vi "main_120MHz.vi"() -> ()   [LabVIEW 2010]
uses:
  <vilib>/Platform/TimedLoop/XDataNode/XDataNode.xnode
  <vilib>/Platform/TimedLoop/XDataNode/nitl_modes.ctl
  <vilib>/Platform/TimedLoop/XDataNode/XDNodeRunTimeDep.lvlib
  <vilib>/Platform/TimedLoop/XDataNode/wakeup.ctl
  <vilib>/Platform/TimedLoop/XDataNode/timing_clust.ctl
  <vilib>/eio/EIONode/EIONode.xnode
  common_typedefs/channels_cluster.ctl
  common_typedefs/gate_parameters_cluster.ctl
panel:
  in  "clamp first pixel?":bool
  in  "gate 3":T1
  in  "gate 2":T1
  in  "gate 1":T1
  out "integrated pixel values":T2
  out "data read":T2
  in  "channel offsets":T2
  out "clock 3 state":bool
  out "clock 2 state":bool
  out "clock 1 state":bool
  in  "stop acquisition at FIFO overflow?":bool=TRUE
  in  "wait for trigger?":bool
  in  "stop":bool
  in  "acquire":bool
  out "acquiring?":bool
  out "FIFO overflow":bool
  out "current pixel no.":i64
  in  "number of pixels":i64=-1
  in  "maximum bit depth":i8
  in  "iterations per pixel":u32
  in  "enable ADC clock?":bool=TRUE
  in  "ADC clock phase":u8
  in  "converter box version":i16=1 min=1 max=2
  # "Outputs / displays"
  # "Integration parameters"
  # "Clock parameters"
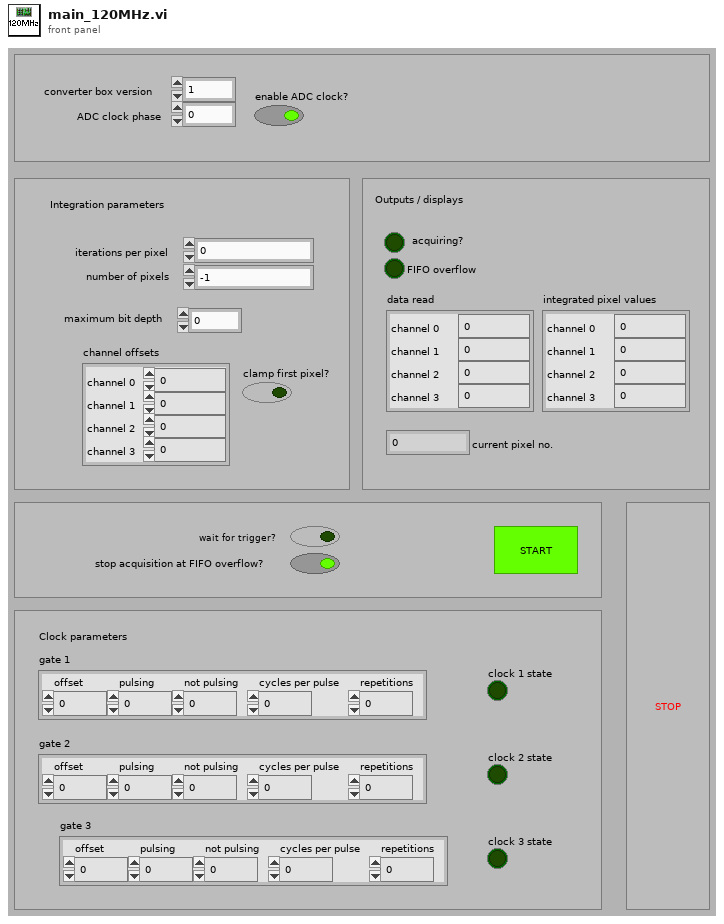
[diagram p1: front panel]
types:
  T1 = typedef "gate_parameters_cluster.ctl" = cluster{"offset":i64, "pulsing":i64, "not pulsing":i64, "cycles per pulse":i64, "repetitions":i64}
  T2 = typedef "channels_cluster.ctl" = cluster{"channel 0":u32, "channel 1":u32, "channel 2":u32, "channel 3":u32}
  T3 = typedef "XDNodeRunTimeDep.lvlib/timing_clust.ctl" = cluster{"Expected End [f-1]":u64, "Actual End [f-1]":u64, "Finished Late? [f-1]":bool, "Expected End [i-1]":u64, "Actual End [i-1]":u64, "Finished Late? [i-1]":bool, "Expected Start [i]":u64, "Actual Start [i]":u64, "Expected Start [f]":u64, "Actual Start [f]":u64, "Source Name":string, "Structure Name":string, "Period":i64, "Deadline":i64, "Offset":i64, "Start":i64, "Priority":i32, "Timeout":i32, "Mode":T4, "Wakeup Reason":T5, "Error":errorcluster, "Source Type":string, "Secondary Source Type":string, "Global End Time":u64, "Global Start Time":u64, "Frame Duration":u64, "Iteration Duration":u64, "Assigned CPU":i32, "I/O Scan Engine Mode":u32}
  T4 = typedef "XDNodeRunTimeDep.lvlib/nitl_modes.ctl" = enum32{"No Change", "Process missed periods, maintain original phase", "Discard missed periods, maintain original phase", "Process missed periods, ignore original phase", "Discard missed periods, ignore original phase"}
  T5 = typedef "XDNodeRunTimeDep.lvlib/wakeup.ctl" = enum32{"Normal", "Aborted", "Asynchronous wakeup", "Timing source error", "Timed loop error", "Timeout"}
  T6 = typedef "gate_counters_cluster.ctl" = cluster{"phase iteration counter":i64, "phase repetition counter":i64, "pulse iteration counter":i64, "phase state":bool}
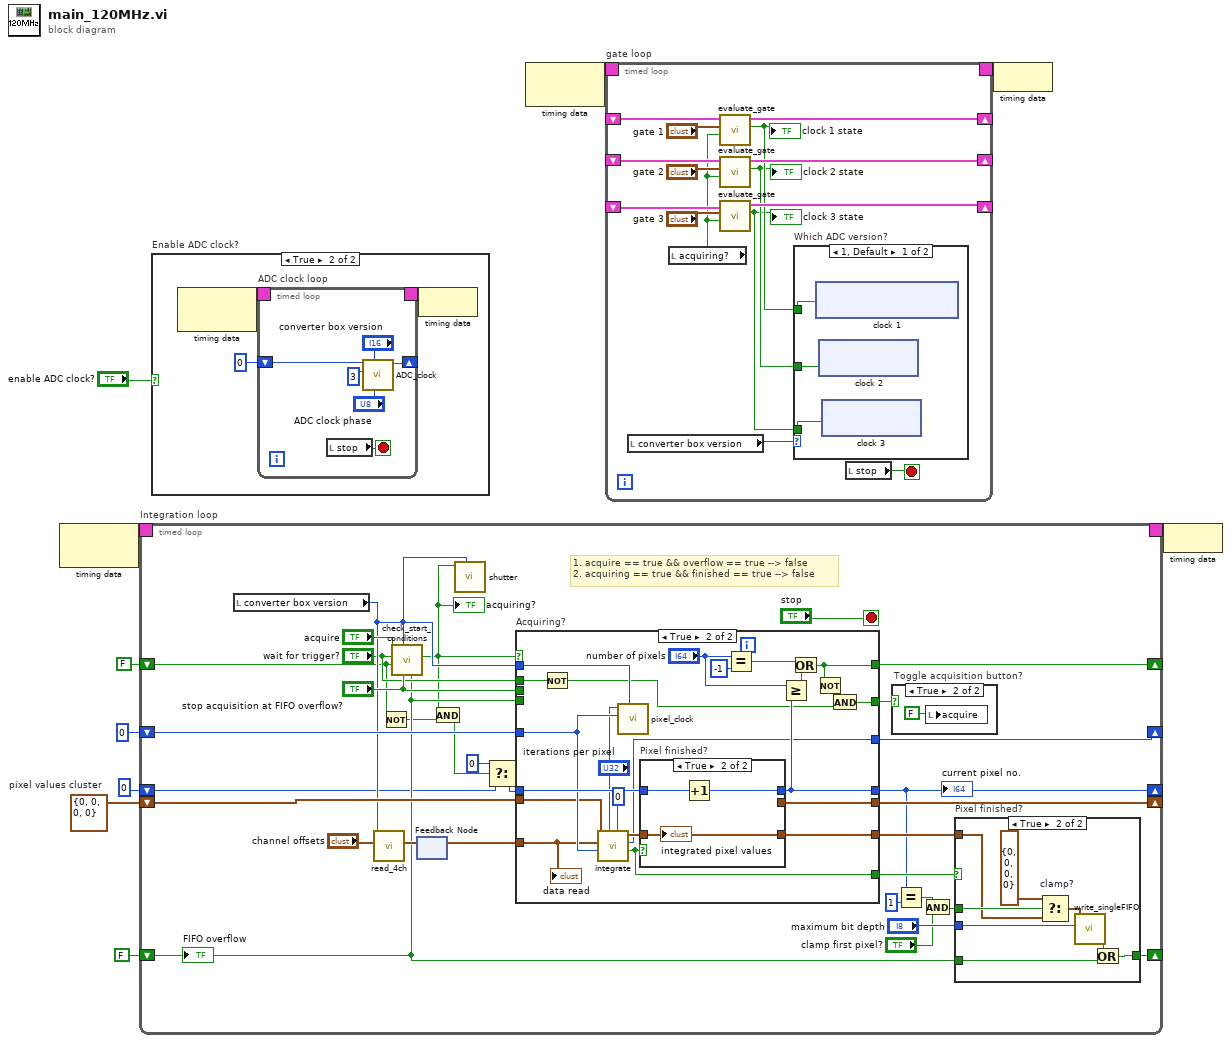
[diagram p0: block diagram]
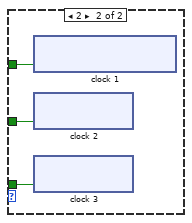
[diagram p2: hidden frame]
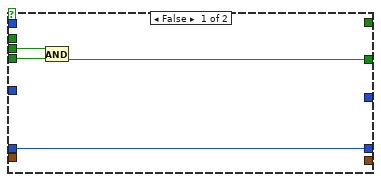
[diagram p5: hidden frame]
diagram:
  w4 = T2 {"channel 0"=0, "channel 1"=0, "channel 2"=0, "channel 3"=0}  # pixel values cluster
  n1 = node-c288() -> (w9:T3)  [unwired: 1 in]
  n2 = timed-loop "Integration loop" {
    timing: w9 -> [_]
    timing-out: [_] -> w8
    shift-right: [w18] -> _
    shift-left: i64 0 -> [w16]
    shift-right: [w36] -> _
    shift-left: u32 0 ("iteration counter out") -> [w38]
    shift-right: [w37] -> _
    shift-left: w4 -> [w39]
    shift-right: [w27] -> _
    shift-left: FALSE -> [w26]
    shift-right: [w31] -> _
    shift-left: FALSE -> [w12]
    stop <- "stop" stop-if-true
    # "1. acquire == true && overflow == true --> false\n2. acquiring == true && finished == true --> false"
    n3 = local read "converter box version"() -> (w30:i16)
    n4 = call "read_4ch.vi"("channel offsets"="channel offsets", "converter box version"=w30) -> ("read output"=w34:T2)  [unwired: 9 in]
    n5 = Not(x=w12) -> (.not. x?=w13:bool)
    n6 = call "check_start_conditions.vi"("FIFO overflow?"=w26, "stop at FIFO overflow?"="stop acquisition at FIFO overflow?", "converter box version"=w30, "already acquiring?"=w12, "in triggered mode?"="wait for trigger?", "acquire"="acquire") -> ("acquire?"=w11:bool)  [unwired: 5 in]
    "acquiring?" <- w11
    n7 = feedback-in #1(w34) -> ()
    n8 = feedback #1() -> (w33:T2)  [unwired: 1 in]
    n9 = And(x=w11, y=w13) -> (x .and. y?=w14:bool)
    n10 = call "shutter.vi"("converter box version"=w30, "open?"=w11) -> ()  [unwired: 10 in]
    n11 = Select(t=i64 0, s=w14, f=w16) -> (s? t:f=w15:i64)
    n12 = case "Acquiring?" shown="True" w11 {
      tunnel: w30 -> [_ w77]
      tunnel: [_ w63] -> w25
      tunnel: [_ w69] -> w36
      tunnel: [w52 w73] -> w18
      tunnel: w39 -> [_ w66]
      tunnel: w15 -> [w52 w71]
      tunnel: w38 -> [_ w68]
      tunnel: [_ w72] -> w37
      tunnel: w33 -> [_ w67]
      tunnel: "stop acquisition at FIFO overflow?" -> [w55 _]
      tunnel: [_ w61] -> w31
      tunnel: [w53 w58] -> w28
      tunnel: w26 -> [w54 _]
      tunnel: "wait for trigger?" -> [_ w60]
      tunnel: [_ w56] -> w24
      frame False {
        n13 = And(x=w54, y=w55) -> (x .and. y?=w53:bool)
      }
      frame True {
        n14 = Not(x=w60) -> (.not. x?=w57:bool)
        n15 = call "integrate.vi"("waiting iterations per pixel"=u32 0, "integration iterations per pixel"="iterations per pixel", "iteration counter in"=w68, "sampling values in"=w67, "previous pixel values in"=w66) -> ("finished?"=w56:bool, "iteration counter out"=w69:u32, "new pixel values out"=w70:T2)  [unwired: 4 in]
        n16 = call "pixel_clock.vi"("converter box version"=w77, "current iteration"=w68, "iterations per pixel"="iterations per pixel") -> ()  [unwired: 9 in]
        n17 = case "Pixel finished?" shown="True" w56 {
          tunnel: w70 -> [w79 w82]
          tunnel: [_ w82] -> w63
          tunnel: [w78 w80] -> w73
          tunnel: w71 -> [w78 w81]
          tunnel: [w79 _] -> w72
          frame False {
          }
          frame True {
            n18 = Increment(x=w81) -> (x+1=w80:i64)
            "integrated pixel values" <- w82
          }
        }
        n19 = Equal?(x="number of pixels", y=i64 -1 ("x")) -> (x = y?=w76:bool)
        n20 = Greater Or Equal?(x="number of pixels", y=w73) -> (x >= y?=w75:bool)
        n21 = Or(x=w76, y=w75) -> (x .or. y?=w61:bool)
        n22 = Not(x=w61) -> (.not. x?=w59:bool)
        n23 = And(x=w59, y=w57) -> (x .and. y?=w58:bool)
        "data read" <- w67
      }
    }
    "current pixel no." <- w18
    n24 = case "Toggle acquisition button?" shown="True" w28 {
      frame False {
      }
      frame True {
        n25 = local write "acquire"(FALSE) -> ()
      }
    }
    n26 = Equal?(x=w18, y=i64 1) -> (x = y?=w21:bool)
    n27 = And(x=w21, y="clamp first pixel?") -> (x .and. y?=w20:bool)
    n28 = case "Pixel finished?" shown="True" w24 {
      tunnel: w25 -> [_ w45]
      tunnel: [w42 w48] -> w27
      tunnel: w26 -> [w42 w47]
      tunnel: "maximum bit depth" -> [_ w50]
      tunnel: w20 -> [_ w46]
      frame False {
      }
      frame True {
        n29 = Select "clamp?"(t=T2 {"channel 0"=0, "channel 1"=0, "channel 2"=0, "channel 3"=0}, s=w46, f=w45) -> (s? t:f=w44:T2)
        n30 = call "write_singleFIFO.vi"("maximum bit depth"=w50, "values to be written"=w44) -> ("FIFO overflow"=w49:bool)  [unwired: 9 in]
        n31 = Or(x=w49, y=w47) -> (x .or. y?=w48:bool)
      }
    }
    "FIFO overflow" <- w26
  }
  n32 = case "Enable ADC clock?" shown="True" "enable ADC clock?" {
    frame False {
    }
    frame True {
      n33 = node-c288() -> (w87:T3)  [unwired: 1 in]
      n34 = timed-loop "ADC clock loop" {
        timing: w87 -> [_]
        timing-out: [_] -> w86
        shift-right: [w92] -> _
        shift-left: u8 0 ("counter out") -> [w93]
        stop <- w89 stop-if-true
        n35 = local read "stop"() -> (w89:bool)
        n36 = call "ADC_clock.vi"("phase"="ADC clock phase", "converter box version"="converter box version", "iterations per cycle"=u8 3, "counter in"=w93) -> ("counter out"=w92:u8)  [unwired: 7 in]
      }
      n37 = node-c288(w86) -> ()
    }
  }
  n38 = node-c288() -> (w3:T3)  [unwired: 1 in]
  n39 = timed-loop "gate loop" {
    timing: w3 -> [_]
    timing-out: [_] -> w2
    shift-right: [w111] -> _
    shift-left: _ -> [w112]
    shift-right: [w109] -> _
    shift-left: _ -> [w110]
    shift-right: [w108] -> _
    shift-left: _ -> [w107]
    stop <- w102 stop-if-true
    n40 = local read "converter box version"() -> (w101:i16)
    n41 = local read "acquiring?"() -> (w103:bool)
    n42 = call "evaluate_gate.vi"("acquiring?"=w103, "gate settings"="gate 1", "gate counters in"=w112) -> ("pulse state out"=w100:bool, "gate counters out"=w111:T6)  [unwired: 7 in]
    "clock 1 state" <- w100
    n43 = call "evaluate_gate.vi"("acquiring?"=w103, "gate settings"="gate 2", "gate counters in"=w110) -> ("pulse state out"=w99:bool, "gate counters out"=w109:T6)  [unwired: 7 in]
    "clock 2 state" <- w99
    n44 = call "evaluate_gate.vi"("acquiring?"=w103, "gate settings"="gate 3", "gate counters in"=w107) -> ("pulse state out"=w98:bool, "gate counters out"=w108:T6)  [unwired: 7 in]
    "clock 3 state" <- w98
    n45 = case "Which ADC version?" shown="1, Default" w101 {
      tunnel: w100 -> [w113 w118]
      tunnel: w99 -> [w114 w117]
      tunnel: w98 -> [w115 w116]
      frame 1, Default {
        n46 = xnode "clock 1"("Connector1/DIO32"=w113) -> ()  [unwired: 1 in, 1 out]
        n47 = xnode "clock 2"("PXI_RTSI_1"=w114) -> ()  [unwired: 1 in, 1 out]
        n48 = xnode "clock 3"("PXI_RTSI_2"=w115) -> ()  [unwired: 1 in, 1 out]
      }
      frame 2 {
        n49 = xnode "clock 1"("Connector0/DIO38"=w118) -> ()  [unwired: 1 in, 1 out]
        n50 = xnode "clock 2"("PXI_RTSI_1"=w117) -> ()  [unwired: 1 in, 1 out]
        n51 = xnode "clock 3"("PXI_RTSI_2"=w116) -> ()  [unwired: 1 in, 1 out]
      }
    }
    n52 = local read "stop"() -> (w102:bool)
  }
  n53 = node-c288(w2) -> ()
  n54 = node-c288(w8) -> ()
